vi "Node - Create Imported Channels.vi"(8 "error in (no error)":errorcluster, 10 "Node Ptr In":T15 format="%.0x", 11 "Compiled.Settings In":T1) -> (0 "error out":errorcluster, 2 "Node Ptr Out":T15=18446744073709551615 format="%.0x", 3 "Compiled.Settings Out":T1)   [LabVIEW 2016, in "PXImc Custom Device System Explorer.lvlib"]
uses:
  PXImc Custom Device System Explorer.lvlib
  <vilib>/NI Veristand/Custom Device API/Custom Device Item Ref.ctl
  Shared/Compiled.Settings.ctl
  <vilib>/NI Veristand/VeriStand Data/Byte Buffer/Byte Buffer.lvclass
  PXImc Router/Controls/Target Type.ctl
  PXImc Router/Controls/Router - Configuration.ctl
  PXImc Router/Controls/Router/Node Block R-W Properties.ctl
  PXImc Router/Controls/Router/Block Properties.ctl
  PXImc Router/Controls/Router/Router - PXImc Properties.ctl
  PXImc Router/Controls/Router/Router - PXImc Card Properties.ctl
  PXImc Router/Controls/Node Data.ctl
  PXImc Router/Controls/Node/Node - PXImc Parameters.ctl
  PXImc Router/Controls/Node/Node - Writer Data.ctl
  PXImc Router/Controls/Node/Node Ch Properties.ctl
  PXImc Router/Controls/Data Type.ctl
  PXImc Router/Controls/Node/Node - Readers Data.ctl
  PXImc Router/Controls/Node/Node - Reader Data.ctl
  <vilib>/NI Veristand/Custom Device API/Custom Device Channel.ctl
  <vilib>/NI Veristand/Custom Device API/Custom Device Channel Type.ctl
  Shared/Constants.vi
  <vilib>/NI VeriStand/Custom Device API/Custom Device API.lvlib
  Shared/PXImc Custom Device Shared.lvlib
  PXImc Router/PXImc Router.lvlib
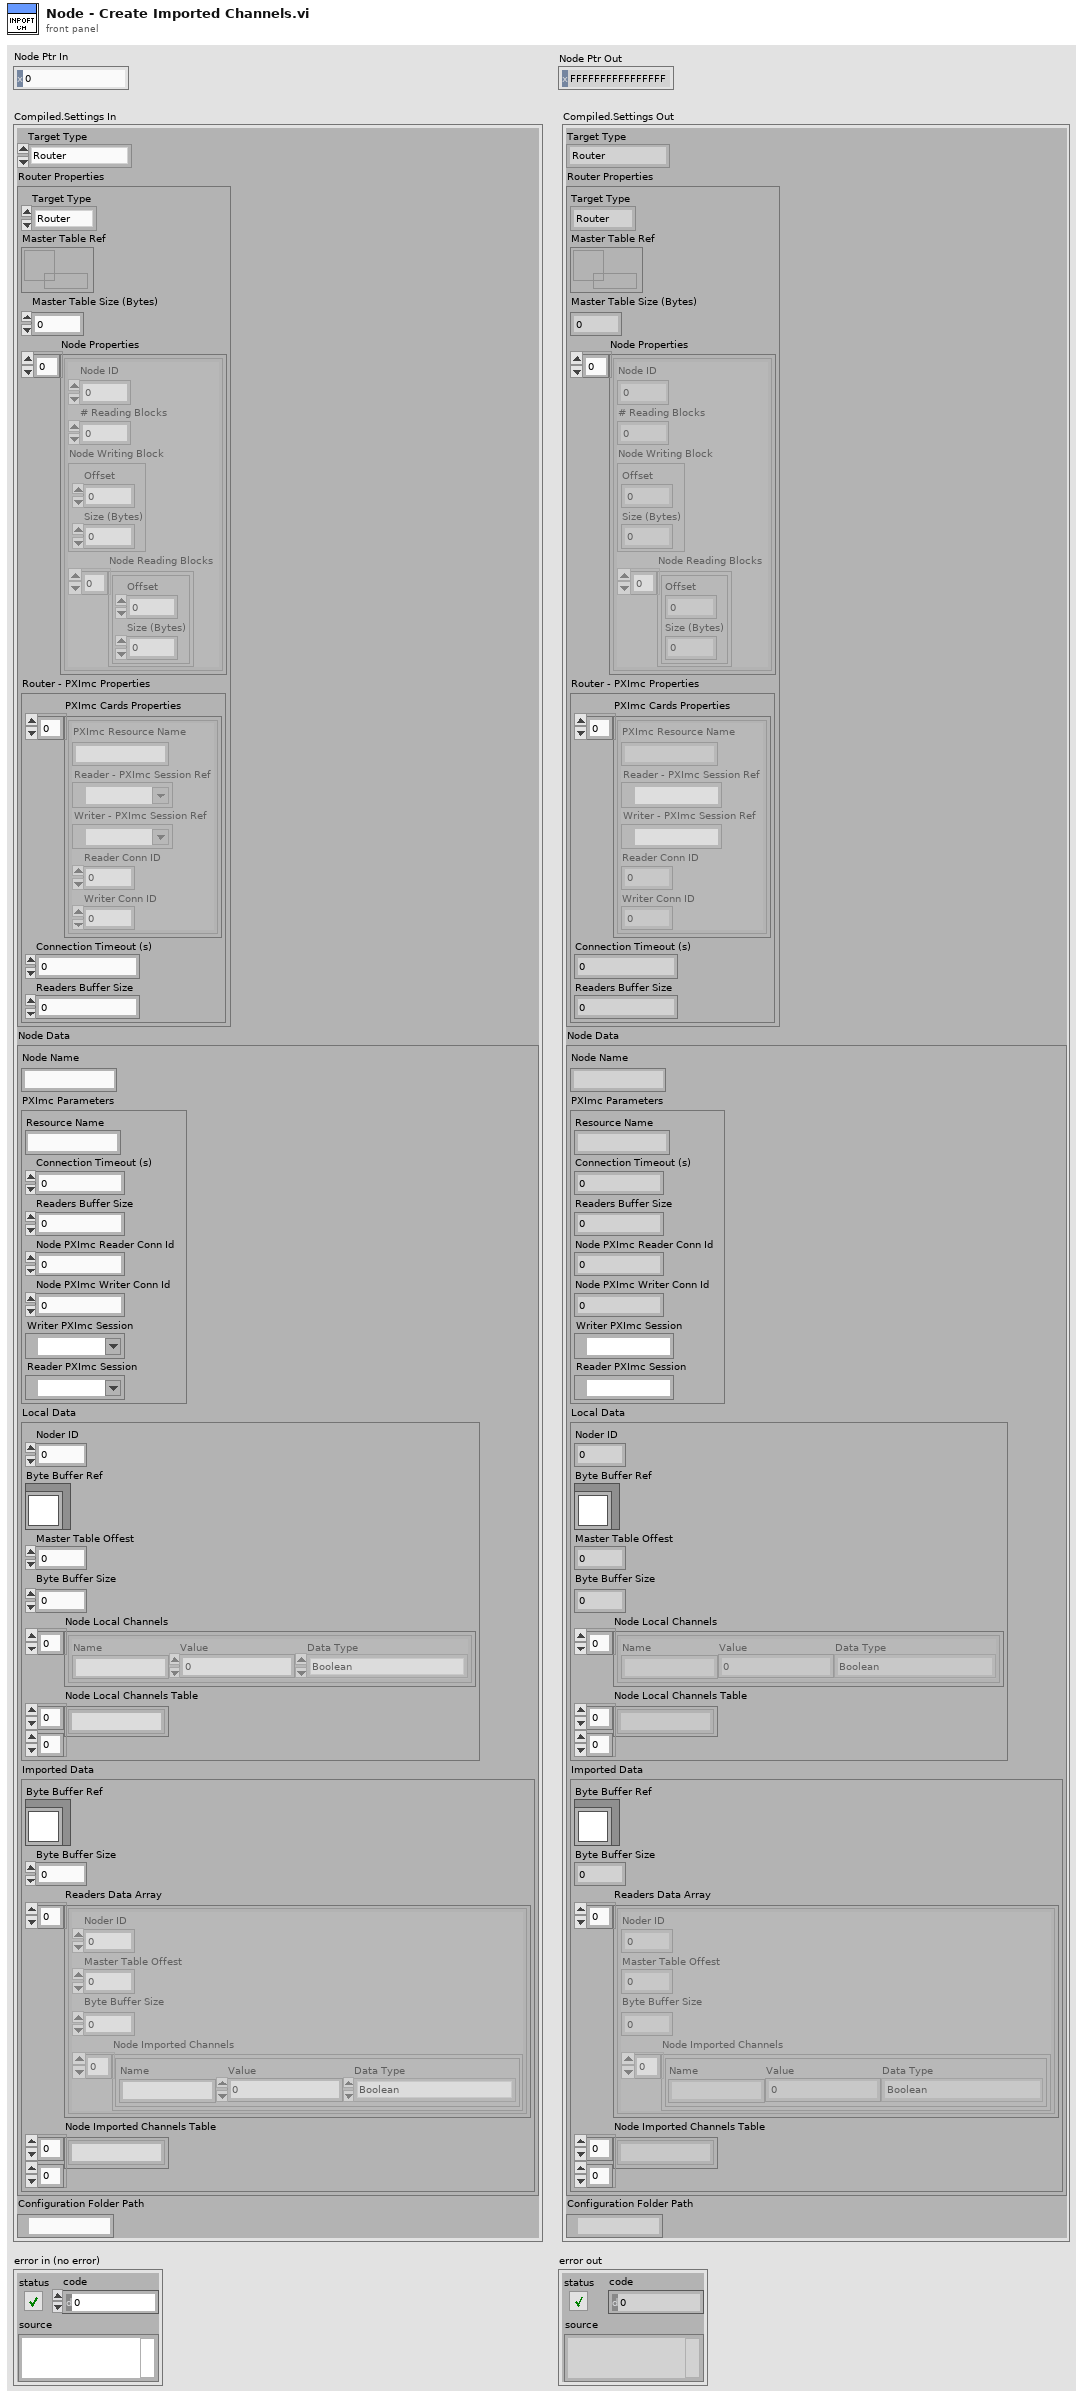
[diagram p1: front panel]
types:
  T1 = typedef "PXImc Custom Device Shared.lvlib/Compiled.Settings.ctl" = cluster{"Target Type":T2, "Router Properties":T3, "Node Data":T8, "Configuration Folder Path":path}
  T2 = typedef "PXImc Router.lvlib/Target Type.ctl" = enum16{"Router", "Node"}
  T3 = typedef "PXImc Router.lvlib/Router - Configuration.ctl" = cluster{"Target Type":T2, "Master Table Ref":refnum<data-value>, "Master Table Size (Bytes)":u32, "Node Properties":T4[], "Router - PXImc Properties":T6}
  T4 = typedef "PXImc Router.lvlib/Node Block R-W Properties.ctl" = cluster{"Node ID":u32, "# Reading Blocks":u32, "Node Writing Block":T5, "Node Reading Blocks":T5[]}
  T5 = typedef "PXImc Router.lvlib/Block Properties.ctl" = cluster{"Offset":u32, "Size (Bytes)":u32}
  T6 = typedef "PXImc Router.lvlib/Router - PXImc Properties.ctl" = cluster{"PXImc Cards Properties":T7[], "Connection Timeout (s)":dbl, "Readers Buffer Size":u64}
  T7 = typedef "PXImc Router.lvlib/Router - PXImc Card Properties.ctl" = cluster{"PXImc Resource Name":string, "Reader - PXImc Session Ref":refnum<k21>, "Writer - PXImc Session Ref":refnum<k21>, "Reader Conn ID":u16, "Writer Conn ID":u16}
  T8 = typedef "PXImc Router.lvlib/Node Data.ctl" = cluster{"Node Name":string, "PXImc Parameters":T9, "Local Data":T10, "Imported Data":T13}
  T9 = typedef "PXImc Router.lvlib/Node - PXImc Parameters.ctl" = cluster{"Resource Name":string, "Connection Timeout (s)":dbl, "Readers Buffer Size":u64, "Node PXImc Reader Conn Id":u16, "Node PXImc Writer Conn Id":u16, "Writer PXImc Session":refnum<k21>, "Reader PXImc Session":refnum<k21>}
  T10 = typedef "PXImc Router.lvlib/Node - Writer Data.ctl" = cluster{"Noder ID":u32, "Byte Buffer Ref":refnum<class "Byte Buffer.lvclass">, "Master Table Offest":u32, "Byte Buffer Size":u32, "Node Local Channels":T11[], "Node Local Channels Table":string[][]}
  T11 = typedef "PXImc Router.lvlib/Node Ch Properties.ctl" = cluster{"Name":string, "Value":dbl, "Data Type":T12}
  T12 = typedef "PXImc Router.lvlib/Data Type.ctl" = enum16{"Boolean", "SGL", "DBL", "I8", "I16", "I32", "I64", "U8", "U16", "U32", "U64"}
  T13 = typedef "PXImc Router.lvlib/Node - Readers Data.ctl" = cluster{"Byte Buffer Ref":refnum<class "Byte Buffer.lvclass">, "Byte Buffer Size":u64, "Readers Data Array":T14[], "Node Imported Channels Table":string[][]}
  T14 = typedef "PXImc Router.lvlib/Node - Reader Data.ctl" = cluster{"Noder ID":u32, "Master Table Offest":u32, "Byte Buffer Size":u64, "Node Imported Channels":T11[]}
  T15 = typedef "Custom Device API.lvlib/Custom Device Item Ref.ctl" = u64
  T16 = typedef "Custom Device API.lvlib/Custom Device Channel.ctl" = cluster{"Type":T17, "Units":string, "Default Value":dbl, "Faultable":bool, "Scalable":bool}
  T17 = typedef "Custom Device API.lvlib/Custom Device Channel Type.ctl" = enum16{"Input", "Output"}
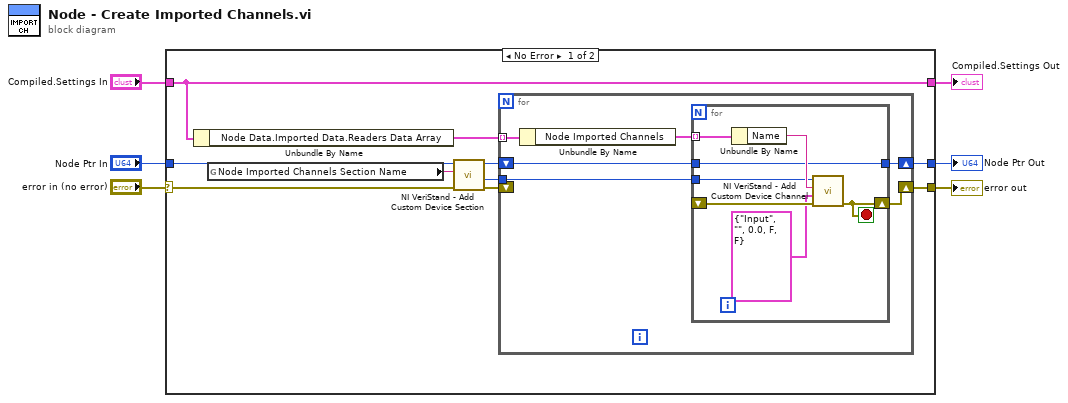
[diagram p0: block diagram]
diagram:
  n1 = case shown="No Error" "error in (no error)" {
    selector: "error in (no error)" -> [w9 w32]
    tunnel: [w16 w32] -> w5
    tunnel: "Node Ptr In" -> [w12 w31]
    tunnel: "Compiled.Settings In" -> [w13 w30]
    tunnel: [w14 w31] -> w2
    tunnel: [w13 w30] -> w1
    frame No Error {
      n2 = Unbundle By Name(w13) -> ("Node Data.Imported Data.Readers Data Array"=w15:T14[])
      n3 = global read "Constants.vi" "Node Imported Channels Section Name"() -> (w7:string)
      n4 = call <vilib>:"NI VeriStand - Add Custom Device Section.vi"("error in (no error)"=w9, "Section Name"=w7, "Parent Ref in"=w12) -> ("error out"=w8:errorcluster, "Section Ptr"=w10:T15, "Parent Ref out"=w11:T15)  [unwired: 5 in, 1 out]
      n5 = for {
        tunnel: w15 -> [w20] mode=indexing
        shift-right: [w21] -> w14
        shift-left: w11 -> [w17]
        shift-right: [w22] -> w16
        shift-left: w8 -> [_]
        tunnel: w10 -> [w18]
        n6 = Unbundle By Name(w20) -> ("Node Imported Channels"=w19:T11[])
        n7 = for {
          shift-right: [w26] -> w22
          shift-left: _ -> [w29]
          tunnel: w17 -> [w23]
          tunnel: w19 -> [w28] mode=indexing
          tunnel: [w23] -> w21
          tunnel: w18 -> [w24]
          stop <- w26 stop-if-true
          n8 = Unbundle By Name(w28) -> ("Name"=w27:string)
          n9 = call <vilib>:"NI VeriStand - Add Custom Device Channel.vi"("error in (no error)"=w29, "Channel"=T16 {"Type"=enum."Input", "Units"="", "Default Value"=0.0, "Faultable"=FALSE, "Scalable"=FALSE}, "Channel Name"=w27, "Parent Ref in"=w24) -> ("error out"=w26:errorcluster)  [unwired: 4 in, 3 out]
        }
      }
    }
    frame Error {
    }
  }
  "error out" <- w5
  "Node Ptr Out" <- w2
  "Compiled.Settings Out" <- w1
